vi "Untitled 1.vi"() -> ()   [LabVIEW 2020]
uses:
  <vilib>/Math Plots/3D Math Plots/3D Scatter/3D Scatter Datatype/3D Scatter Datatype.lvclass
  <vilib>/Math Plots/3D Math Plots/3D Scatter/3D Scatter Datatype/Public/Plot Helper (Vector).vi
  <vilib>/ErrorRing/Error Ring.xnode
  <vilib>/Utility/error.llb/Error Cluster From Error Code.vi
  <vilib>/Math Plots/3D Math Plots/3D Scatter/3D Scatter XCtrl/3D Scatter.xctl
panel:
  out "element":i8
  out "Index":i32
  out "message":string=" INSTRUCTIONS:\r\rNormal Use:  When using subVIs that incorporate the error in/error out (or error I/O) structure, place this handler where you want to inform the user of an error, typically at the end of the I/O data path, as the last action of the program.  If the error in error? is ERROR, the handler creates a message describing the error and its source.  If the type of dialog = 1 (default), the message is displayed to the user, who can only acknowedge it.  If the type = 2, the user can acknowledge the message or abort execution; aborting a program with active I/O is not recommended.  If the type = 0, no message is displayed; this is used to process the error programmatically, and the error out cluster elements are wired to individual terminals for that reason.  \r\rOther Use:\n\r\nlocal testing.  To test the error code of a subVI or function that does not have the error I/O structure, you can wire its error code and a source string to the local error code and error source inputs.  If error in error? indicates no error and error code is not equal to 0, the local code and source are substituted for the error in values, and error? is set TRUE (ERROR)."
  out "substring":string
  out "number":i32
  out "Metadata":T1
  in  "file (use dialog)":path=path "C:/Users/Lexa/DevProjects/Prometheus/Scalable packed voxel mapping/test.spvm"
  out "File data":string
  in  "Slow?":bool=TRUE
  out "Current ring":i32
  in  "Rings to render":i32=24
  out "Ring position":i32
  out "Ring size":i32
  out "3D Scatter":refnum<class "3D Plot Datatype.lvclass">[](xcontrol)
  out "Current position":i8[](array[numeric])
  out "Current vector":i8[](array[numeric])
  out "Next Vector":i32
  out "Vertices ( Cartesian )":dbl[][](array[numeric])
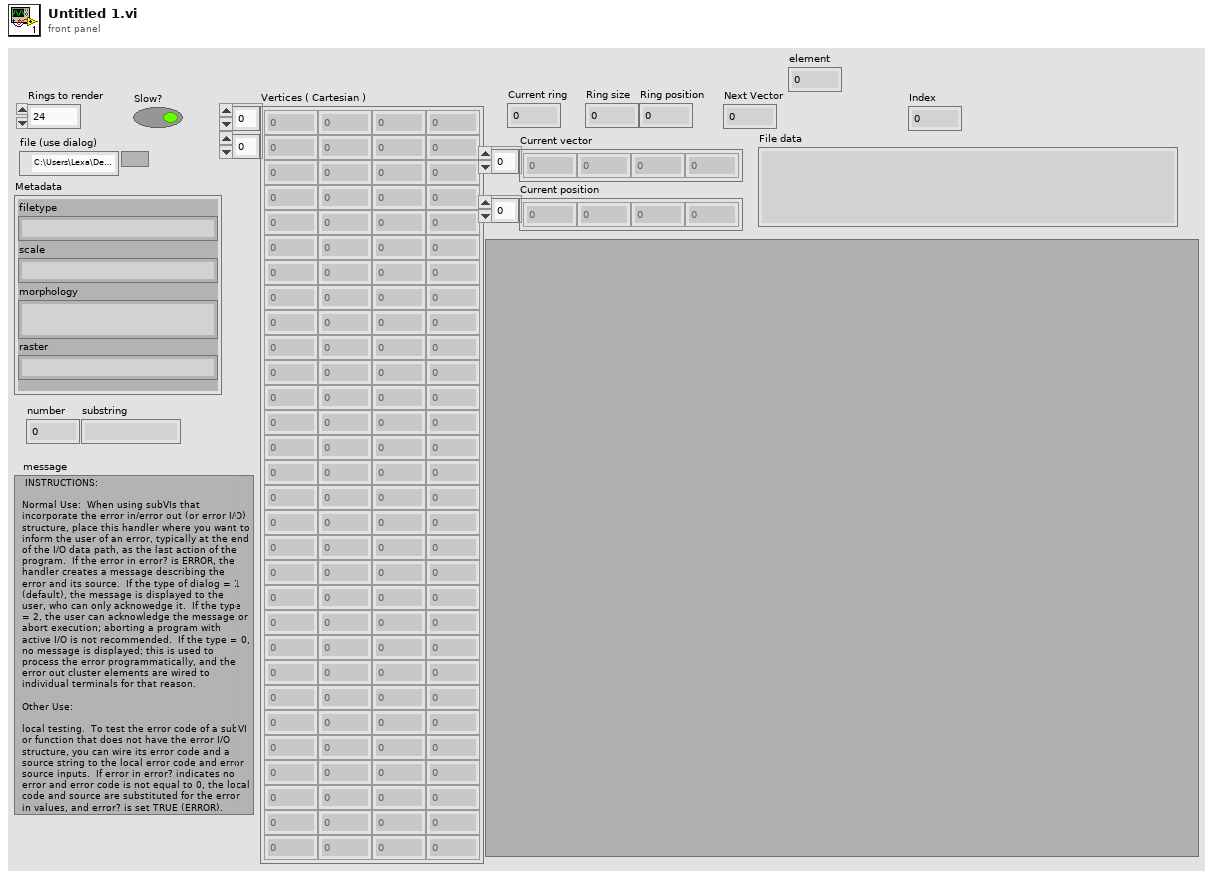
[diagram p1: front panel]
types:
  T1 = cluster{"filetype":string, "scale":string, "morphology":string, "raster":string}
  T2 = cluster{"Filetype":string, "Scale ( µm )":ext, "Morphology":string, "Raster":string, "VectorOrder":string}
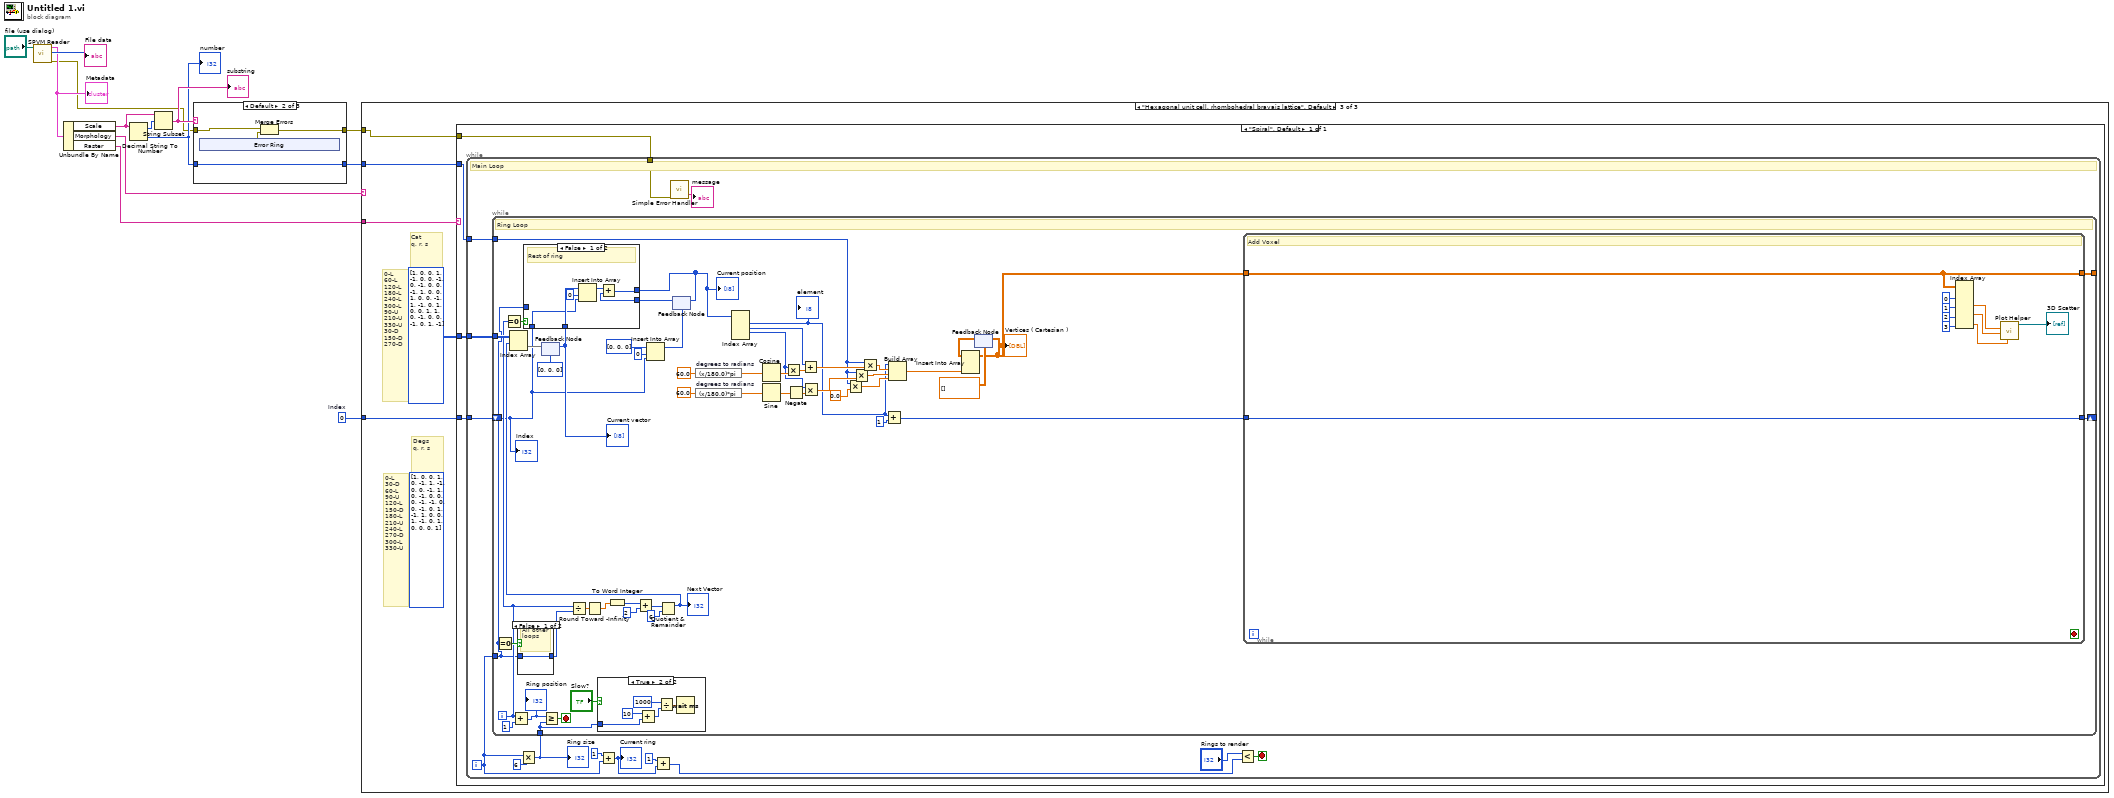
[diagram p0: block diagram]
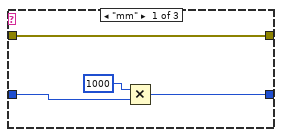
[diagram p2: hidden frame]
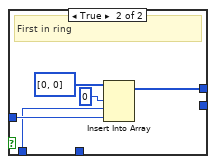
[diagram p7: hidden frame]
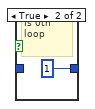
[diagram p8: hidden frame]
diagram:
  w1 = 0  # Index
  n1 = call "SPVM Reader.vi"("file (use dialog)"="file (use dialog)") -> ("error out"=w3:errorcluster, "VoxelData"=→"File data":u8[], "Metadata"=w9:T2)  [unwired: 6 in, 2 out]
  "Metadata" <- w9
  n2 = Unbundle By Name(w9) -> ("Scale"=w7:string, "Morphology"=w11:string, "Raster"=w10:string)
  n3 = Decimal String To Number(string=w7) -> (offset past number=w8:i32, number=w4:i32)  [unwired: 2 in]
  "number" <- w4
  n4 = String Subset(string=w7, offset (0)=w8) -> (substring=w6:string)  [unwired: 1 in]
  "substring" <- w6
  n5 = case shown="Default" w6 {
    tunnel: [w17 w21 w28] -> w5
    tunnel: w4 -> [w16 w21 w28]
    tunnel: w3 -> [w14 w19 w27]
    tunnel: [w14 w20 w27] -> w2
    frame "mm" {
      n6 = Multiply(x=1000, y=w16) -> (x*y=w17:i32)
    }
    frame Default {
      n7 = xnode "Error Ring"() -> ("error out"=w18:errorcluster)
      n8 = Merge Errors(w19, w18) -> (w20:errorcluster)
    }
    frame "µm" {
    }
  }
  n9 = case shown="\"Hexagonal unit cell, rhombohedral bravais lattice\", Default" w11 {
    tunnel: w10 -> [_ _ w33]
    tunnel: w5 -> [_ _ w32]
    tunnel: w2 -> [_ _ w30]
    tunnel: w1 -> [_ _ w29]
    frame "Cubic" {
    }
    frame "Face centered cubic" {
    }
    frame "Hexagonal unit cell, rhombohedral bravais lattice", Default {
      (unwired) i8[][] [[1, 0, 0], [1, 0, -1], [1, -1, 0], [0, -1, 1], [0, -1, 0], [0, 0, -1], [-1, 0, 0], [-1, 0, 1], [-1, 1, 0], [0, 1, -1], [0, 1, 0], [0, 0, 1]]
      # "0-L\n30-D\n60-L\n90-U\n120-L\n150-D\n180-L\n210-U\n240-L\n270-D\n300-L\n330-U"
      # "Degs \nq, r, s"
      # "0-L\n60-L\n120-L\n180-L\n240-L\n300-L\n90-U\n210-U\n330-U\n30-D\n150-D\n270-D"
      # "Cat \nq, r, s"
      n10 = case shown="\"Spiral\", Default" w33 {
        tunnel: w32 -> [w37]
        tunnel: i8[][] [[1, 0, 0], [1, -1, 0], [0, -1, 0], [-1, 0, 0], [-1, 1, 0], [0, 1, 0], [0, -1, 1], [-1, 0, 1], [0, 0, 1], [1, 0, -1], [0, 0, -1], [0, 1, -1]] -> [w36]
        tunnel: w30 -> [w35]
        tunnel: w29 -> [w34]
        frame "Spiral", Default {
          n11 = while {
            tunnel: w37 -> [w47]
            tunnel: w36 -> [w41]
            tunnel: w35 -> [w39]
            tunnel: w34 -> [w38]
            i -> [w45]
            stop <- w49 stop-if-true
            # "Main Loop"
            n12 = Multiply(x=w45, y=6) -> (x*y=w50:i32)
            "Ring size" <- w50
            n13 = while {
              tunnel: w45 -> [w80]
              tunnel: w50 -> [w66]
              tunnel: w41 -> [w84]
              tunnel: w47 -> [w67]
              shift-right: [w55] -> _
              shift-left: w38 -> [w56]
              tunnel: [w53] -> _
              i -> [w82]
              stop <- w91 stop-if-true
              # "Ring Loop"
              n14 = Equal To 0?(x=w80) -> (x = 0?=w87:bool)
              n15 = Equal To 0?(x=w82) -> (x = 0?=w81:bool)
              n16 = Add(x=w82, y=1) -> (x+y=w89:i32)
              "Ring position" <- w89
              n17 = case shown="False" w87 {
                tunnel: w80 -> [w131 _]
                tunnel: [w131 1] -> w86
                frame False {
                  # "All other loops"
                }
                frame True {
                  # "Is 0th loop"
                }
              }
              n18 = feedback #1(i8[] [0, 0, 0] ("x")) -> (w79:i8[])
              "Current vector" <- w79
              n19 = Greater Or Equal?(x=w89, y=w66) -> (x >= y?=w91:bool)
              n20 = Divide(x=w82, y=w86) -> (x/y=w96:dbl)
              n21 = Round Toward -Infinity(1:w96) -> (0:w95:dbl)
              n22 = case shown="True" "Slow?" {
                tunnel: w66 -> [_ w118]
                frame False {
                }
                frame True {
                  n23 = Add(x=10, y=w118) -> (x+y=w116:i32)
                  n24 = Divide(x=1000, y=w116) -> (x/y=w115:dbl)
                  n25 = Wait (ms)(milliseconds to wait=w115) -> ()  [unwired: 1 out]
                }
              }
              n26 = To Word Integer(number=w95) -> (16bit integer=w93:i16)
              n27 = Add(x=w93, y=2) -> (x+y=w88:i32)
              n28 = Insert Into Array(array=i8[] [0, 0, 0] ("x"), index=0, new element=w56) -> (w58:i8[])
              n29 = Quotient & Remainder(x=w88, y=6) -> (x-y*floor(x/y)=w85:i32)  [unwired: 1 out]
              "Next Vector" <- w85
              n30 = Index Array(array=w84, index (row)=w85) -> (element=w60:i8[])  [unwired: 1 in]
              n31 = feedback-in #1(w60) -> ()
              n32 = feedback #2(w58) -> (w78:i8[])
              n33 = case shown="False" w81 {
                tunnel: w80 -> [_ w127]
                tunnel: w79 -> [w123 _]
                tunnel: [w125 w128] -> w77
                tunnel: w78 -> [w124 _]
                tunnel: w56 -> [w120 w126]
                frame False {
                  # "Rest of ring"
                  n34 = Insert Into Array(array=w123, index=0, new element=w120) -> (w122:i8[])
                  n35 = Add(x=w122, y=w124) -> (x+y=w125:i8[])
                }
                frame True {
                  # "First in ring"
                  n36 = Insert Into Array(array=i8[] [0, 0] ("x"), index=0, new element #1=w126, new element #2=w127) -> (w128:i8[])
                }
              }
              "Current position" <- w77
              n37 = feedback-in #2(w77) -> ()
              n38 = expression code="(x/180.0)*pi" "degrees to radians"(60.0) -> (w103:dbl)
              n39 = expression code="(x/180.0)*pi" "degrees to radians"(60.0) -> (w101:dbl)
              n40 = Index Array(array=w77) -> (element #1=w61:i8, element #2=w63:i8, element #3=w64:i8)  [unwired: 4 in, 1 out]
              "element" <- w61
              n41 = Cosine(x=w103) -> (cos(x)=w100:dbl)
              n42 = Sine(x=w101) -> (sin(x)=w98:dbl)
              n43 = Multiply(x=w64, y=w100) -> (x*y=w99:dbl)
              n44 = Negate(x=w98) -> (-x=w97:dbl)
              n45 = Add(x=w63, y=w99) -> (x+y=w72:dbl)
              n46 = Multiply(x=w64, y=w97) -> (x*y=w69:dbl)
              n47 = Multiply(x=w67, y=0.0 ("element")) -> (x*y=w70:dbl)
              n48 = Multiply(x=w67, y=w69) -> (x*y=w71:dbl)
              n49 = Multiply(x=w67, y=w72) -> (x*y=w73:dbl)
              n50 = Add(x=w61, y=1 ("index (col)")) -> (x+y=w54:i32)
              n51 = Build Array(w61, w73, w71, w70) -> (w76:dbl[])
              n52 = feedback #3(dbl[][] []) -> (w75:dbl[][])
              n53 = Insert Into Array(array=w75, new element=w76) -> (w52:dbl[][])  [unwired: 2 in]
              "Vertices ( Cartesian )" <- w52
              n54 = feedback-in #3(w52) -> ()
              n55 = while {
                tunnel: [w106] -> w55
                tunnel: w54 -> [w106]
                tunnel: [w105] -> w53
                tunnel: w52 -> [w105]
                stop <- _ stop-if-true
                # "Add Voxel"
                n56 = Index Array(array=w105, index (col) #1=0 ("disabled index (col)"), index (col) #2=1 ("index (col)"), index (col) #3=2 ("index (col)"), index (col) #4=3 ("index (col)")) -> (element #2=w114:dbl[], element #3=w113:dbl[], element #4=w112:dbl[])  [unwired: 4 in, 1 out]
                n57 = call-poly <vilib>:"Plot Helper.vi"("z vector"=w112, "y vector"=w113, "x vector"=w114) -> ("3D Plot lvclass Array out"=→"3D Scatter":refnum<class "3D Plot Datatype.lvclass">[])  [unwired: 3 in, 5 out]
              }
              "Index" <- w56
            }
            n58 = Add(x=1, y=w45) -> (x+y=w43:i32)
            "Current ring" <- w43
            n59 = Add(x=1, y=w43) -> (x+y=w42:i32)
            n60 = call <vilib>:"Simple Error Handler.vi"("error in (no error)"=w39) -> ("message"=→"message":string)  [unwired: 4 in, 4 out]
            n61 = Less?(x="Rings to render", y=w42) -> (x < y?=w49:bool)
          }
        }
      }
    }
  }
